vi "Demo- Create and Update Feature Studio in default document.vi"() -> ()   [LabVIEW 2019]
uses:
  _SubVI/default document.vi
panel:
  in  "FeatureScript":string
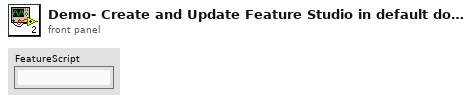
[diagram p1: front panel]
types:
  T1 = typedef "Cluster.ctl" = cluster{"Date":string, "On-Nonce":string, "eid":string, "wid":string, "did":string, "name":string, "method":string, "Accept":string, "User-Agent":string, "Content-Type":string, "stack":string, "headers":string[], "payload":string, "ctype":string, "path":string, "Authorization":string, "secret_key":string, "access_key":string}
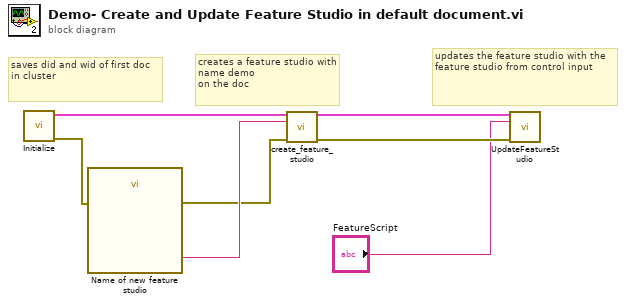
[diagram p0: block diagram]
diagram:
  # "updates the feature studio with the feature studio from control input"
  # "creates a feature studio with name demo\non the doc"
  # "saves did and wid of first doc in cluster"
  n1 = call-poly "Initialize.vi"() -> ("Device Out"=w7:T1, "error out"=w2:errorcluster)  [unwired: 13 in, 1 out]
  n2 = call "Name of new feature studio"("error in (no error)"=w2) -> ("Name"=w3:string, "error out"=w1:errorcluster)  [unwired: 16 in, 1 out]
  n3 = call "create_feature_studio.vi"("Device In"=w7, "New Feature Studio Name"=w3, "error in"=w1) -> ("Device Out"=w6:T1, "error out"=w5:errorcluster)  [unwired: 10 in, 1 out]
  n4 = call "UpdateFeatureStudio.vi"("Device In"=w6, "FeatureScript"="FeatureScript", "error in"=w5) -> ()  [unwired: 10 in, 3 out]
